vi "Shooter Button SUBVI.vi"   [LabVIEW 2011]
types:
  T1 = cluster{"Digital Input [1-16][0]":bool, "Digital Input [1-16][1]":bool, "Digital Input [1-16][2]":bool, "Digital Input [1-16][3]":bool, "Digital Input [1-16][4]":bool, "Digital Input [1-16][5]":bool, "Digital Input [1-16][6]":bool, "Digital Input [1-16][7]":bool, "Digital Input [1-16][8]":bool, "Digital Input [1-16][9]":bool, "Digital Input [1-16][10]":bool, "Digital Input [1-16][11]":bool, "Digital Input [1-16][12]":bool, "Digital Input [1-16][13]":bool, "Digital Input [1-16][14]":bool, "Digital Input [1-16][15]":bool}
  T2 = typedef "WPI_DigitalInputDevRef.ctl" = cluster{"DevStatus":errorcluster, "DIO Channel":T3, "Digital Module":T4}
  T3 = typedef "FPGA_DIOChannel.ctl" = enum8{"DIO 1", "DIO 2", "DIO 3", "DIO 4", "DIO 5", "DIO 6", "DIO 7", "DIO 8", "DIO 9", "DIO 10", "DIO 11", "DIO 12", "DIO 13", "DIO 14", "Invalid"}
  T4 = typedef "FPGA_TypedefDigitalModule.ctl" = enum16{"Digital Module 1", "Digital Module 2"}
  T5 = typedef "WPI_MotorControlDeviceRef.ctl" = cluster{"DeviceStatus":errorcluster, "Type":enum16{"PWM", "CAN"}, "PWM":cluster{"Digital Module":T4, "PWM Channel":T6, "DeadBand":T7}, "CAN":cluster{"Device Number":u8, "Control Mode":T8, "Semaphore":T9, "Max Vout":dbl}, "Invert":bool, "TransformRef":T10, "InvTransformRef":T10}
  T6 = typedef "FPGA_DIOPWMChannel.ctl" = enum8{"PWM 1", "PWM 2", "PWM 3", "PWM 4", "PWM 5", "PWM 6", "PWM 7", "PWM 8", "PWM 9", "PWM 10", "Invalid"}
  T7 = typedef "WPI_PWMDeadband.ctl" = cluster{"Name":string, "maxPositivePwm":i32, "minPositivePwm":i32, "centerPwm":i32, "maxNegativePwm":i32, "minNegativePwm":i32, "angularRange":u16}
  T8 = typedef "WPI_CANJaguar_ControlMode.ctl" = enum8{"Percent VBus", "Current", "Speed", "Position", "Voltage"}
  T9 = typedef "Semaphore RefNum" = refnum<k1>
  T10 = typedef "WPI_PWMTransform_ConPane.ctl" = refnum<vi>
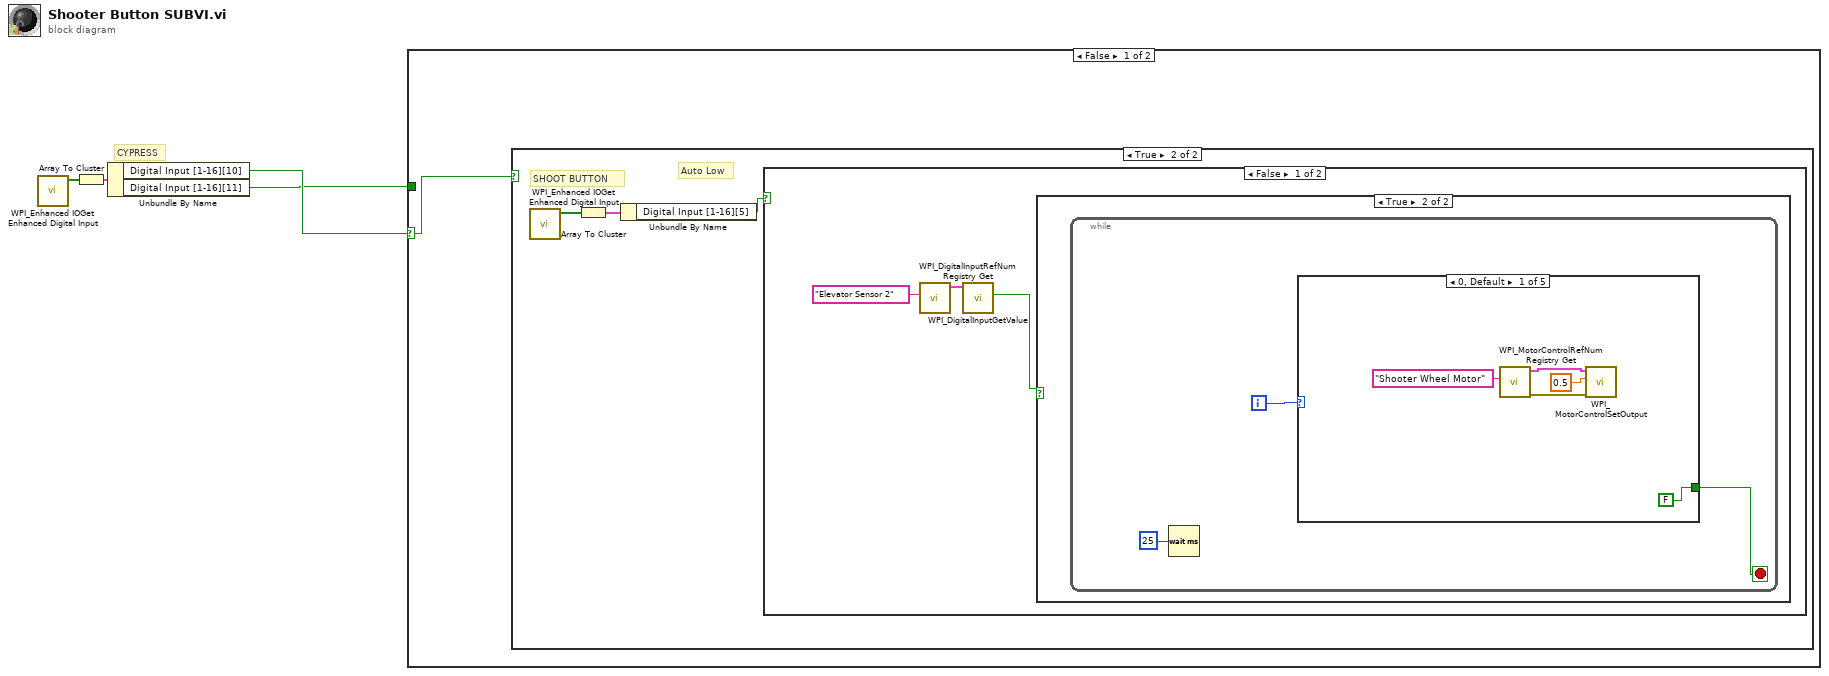
[diagram p0: block diagram]
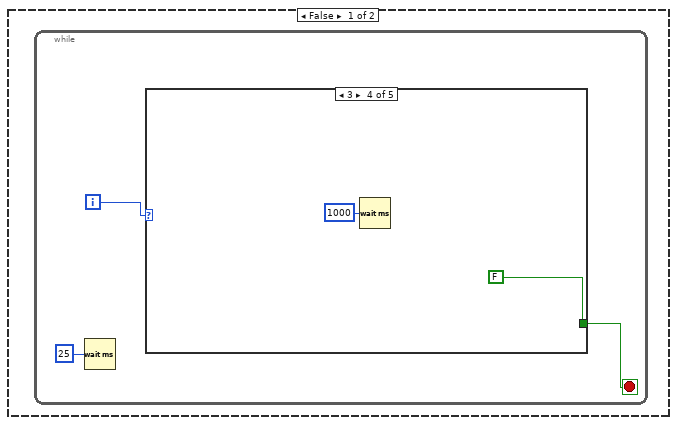
[diagram p3: hidden frame]
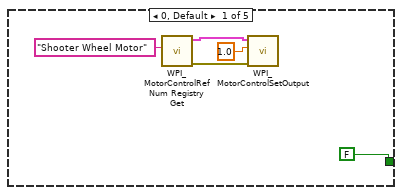
[diagram p4: hidden frame]
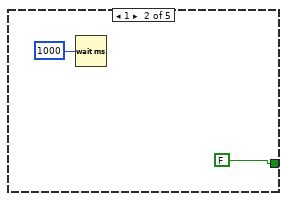
[diagram p5: hidden frame]
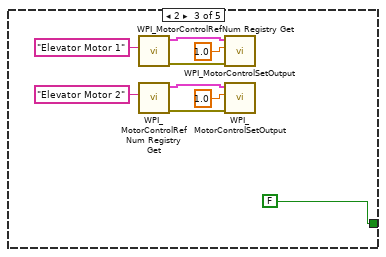
[diagram p6: hidden frame]
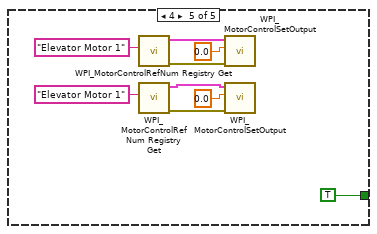
[diagram p7: hidden frame]
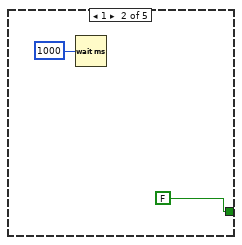
[diagram p8: hidden frame]
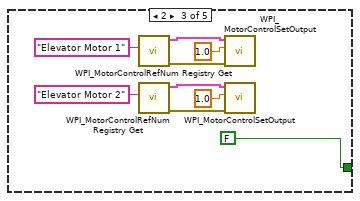
[diagram p9: hidden frame]
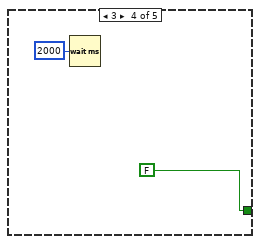
[diagram p10: hidden frame]
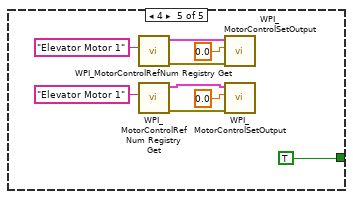
[diagram p11: hidden frame]
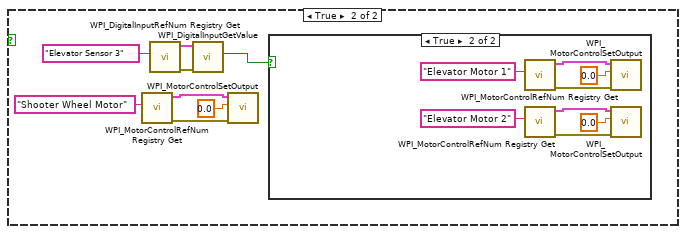
[diagram p12: hidden frame]
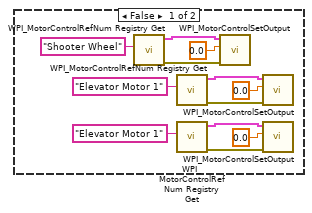
[diagram p13: hidden frame]
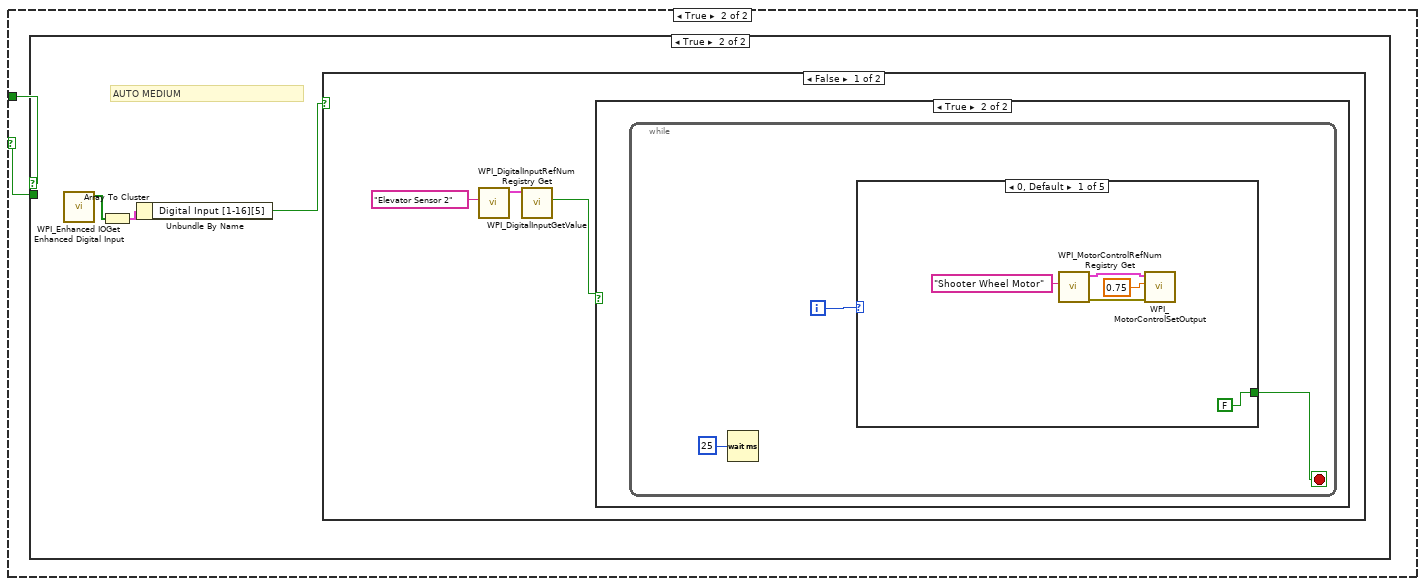
[diagram p14: hidden frame]
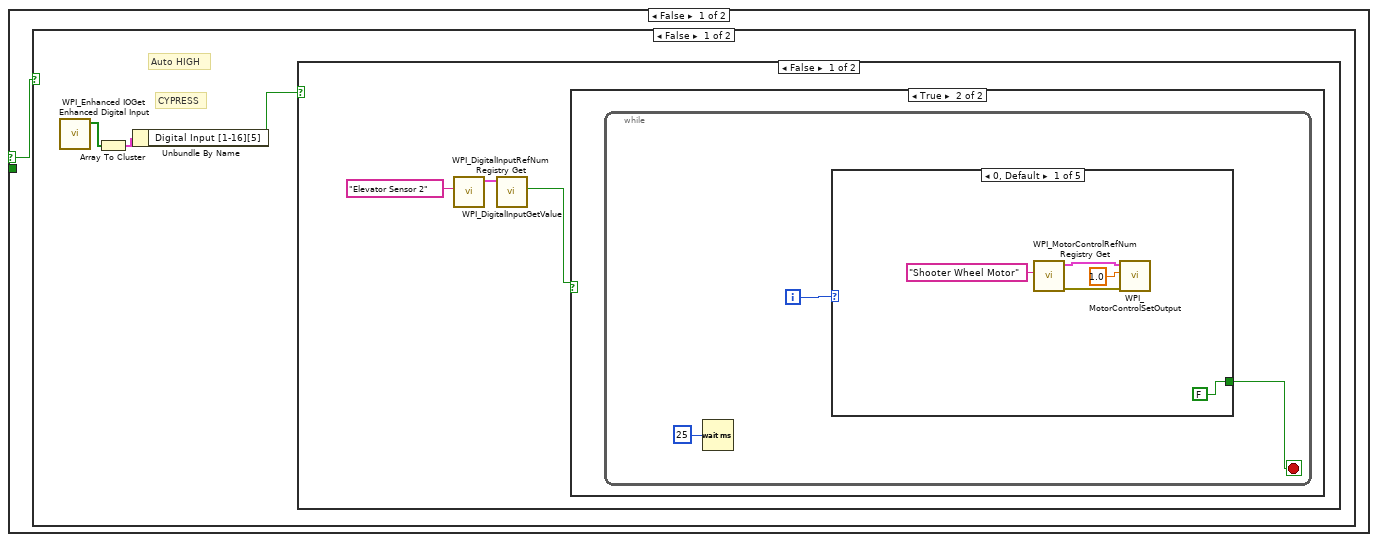
[diagram p15: hidden frame]
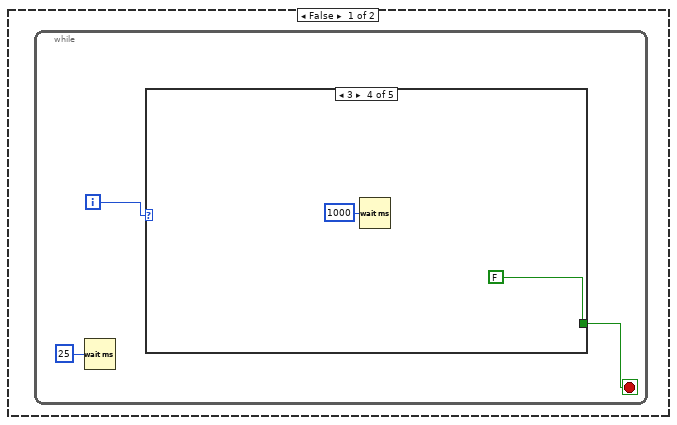
[diagram p16: hidden frame]
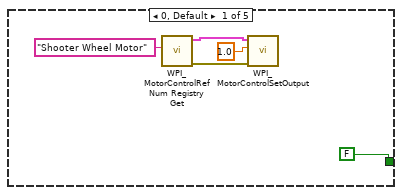
[diagram p17: hidden frame]
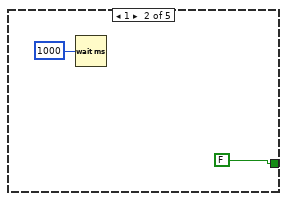
[diagram p18: hidden frame]
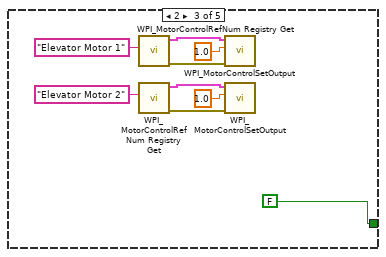
[diagram p19: hidden frame]
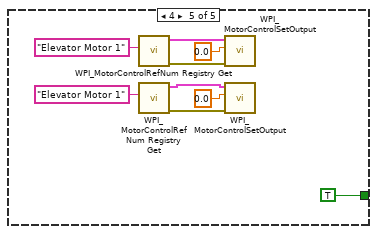
[diagram p20: hidden frame]
diagram:
  # "CYPRESS"
  n1 = call <vilib>:"WPI_Enhanced IOGet Enhanced Digital Input.vi"() -> ("Digital Input [1-16]"=w4:bool[])  [unwired: 10 in, 1 out]
  n2 = Array To Cluster(array=w4) -> (cluster=w3:T1)
  n3 = Unbundle By Name(w3) -> ("Digital Input [1-16][10]"=w2:bool, "Digital Input [1-16][11]"=w1:bool)
  n4 = case shown="False" w2 {
    selector: w2 -> [w5 w100]
    tunnel: w1 -> [_ w101]
    frame False {
      n5 = case shown="True" w5 {
        frame False {
        }
        frame True {
          # "Auto Low"
          # "SHOOT BUTTON"
          n6 = call <vilib>:"WPI_Enhanced IOGet Enhanced Digital Input.vi"() -> ("Digital Input [1-16]"=w8:bool[])  [unwired: 10 in, 1 out]
          n7 = Array To Cluster(array=w8) -> (cluster=w7:T1)
          n8 = Unbundle By Name(w7) -> ("Digital Input [1-16][5]"=w6:bool)
          n9 = case shown="False" w6 {
            frame False {
              n10 = call <vilib>:"WPI_DigitalInputRefNum Registry Get.vi"("refnum name"="Elevator Sensor 2") -> ("DigitalInputDevRef"=w10:T2)  [unwired: 9 in, 1 out]
              n11 = call <vilib>:"WPI_DigitalInputGetValue.vi"("DigitalInputDevRef"=w10) -> ("Value"=w9:bool)  [unwired: 8 in, 2 out]
              n12 = case shown="True" w9 {
                frame False {
                  n13 = while {
                    i -> [w14]
                    stop <- w12 stop-if-true
                    n14 = Wait (ms)(milliseconds to wait=u32 25) -> ()  [unwired: 1 out]
                    n15 = case shown="3" w14 {
                      tunnel: [FALSE FALSE FALSE FALSE TRUE] -> w12
                      frame 0, Default {
                        n16 = call <vilib>:"WPI_MotorControlRefNum Registry Get.vi"("refnum name"="Shooter Wheel Motor") -> ("error out"=w19:errorcluster, "MotorControlDevRef"=w18:T5)  [unwired: 9 in]
                        n17 = call <vilib>:"WPI_MotorControlSetOutput.vi"("error in (no error)"=w19, "Output"=1.0, "MotorControlDevRef"=w18) -> ()  [unwired: 7 in, 2 out]
                      }
                      frame 1 {
                        n18 = Wait (ms)(milliseconds to wait=u32 1000) -> ()  [unwired: 1 out]
                      }
                      frame 2 {
                        n19 = call <vilib>:"WPI_MotorControlRefNum Registry Get.vi"("refnum name"="Elevator Motor 1") -> ("error out"=w26:errorcluster, "MotorControlDevRef"=w25:T5)  [unwired: 9 in]
                        n20 = call <vilib>:"WPI_MotorControlRefNum Registry Get.vi"("refnum name"="Elevator Motor 2") -> ("error out"=w30:errorcluster, "MotorControlDevRef"=w29:T5)  [unwired: 9 in]
                        n21 = call <vilib>:"WPI_MotorControlSetOutput.vi"("error in (no error)"=w26, "Output"=1.0, "MotorControlDevRef"=w25) -> ()  [unwired: 7 in, 2 out]
                        n22 = call <vilib>:"WPI_MotorControlSetOutput.vi"("error in (no error)"=w30, "Output"=1.0, "MotorControlDevRef"=w29) -> ()  [unwired: 7 in, 2 out]
                      }
                      frame 3 {
                        n23 = Wait (ms)(milliseconds to wait=1000) -> ()  [unwired: 1 out]
                      }
                      frame 4 {
                        n24 = call <vilib>:"WPI_MotorControlRefNum Registry Get.vi"("refnum name"="Elevator Motor 1") -> ("error out"=w39:errorcluster, "MotorControlDevRef"=w34:T5)  [unwired: 9 in]
                        n25 = call <vilib>:"WPI_MotorControlRefNum Registry Get.vi"("refnum name"="Elevator Motor 1") -> ("error out"=w35:errorcluster, "MotorControlDevRef"=w36:T5)  [unwired: 9 in]
                        n26 = call <vilib>:"WPI_MotorControlSetOutput.vi"("error in (no error)"=w39, "Output"=0.0, "MotorControlDevRef"=w34) -> ()  [unwired: 7 in, 2 out]
                        n27 = call <vilib>:"WPI_MotorControlSetOutput.vi"("error in (no error)"=w35, "Output"=0.0, "MotorControlDevRef"=w36) -> ()  [unwired: 7 in, 2 out]
                      }
                    }
                  }
                }
                frame True {
                  n28 = while {
                    i -> [w44]
                    stop <- w42 stop-if-true
                    n29 = Wait (ms)(milliseconds to wait=u32 25) -> ()  [unwired: 1 out]
                    n30 = case shown="0, Default" w44 {
                      tunnel: [FALSE FALSE FALSE FALSE TRUE] -> w42
                      frame 0, Default {
                        n31 = call <vilib>:"WPI_MotorControlRefNum Registry Get.vi"("refnum name"="Shooter Wheel Motor") -> ("error out"=w49:errorcluster, "MotorControlDevRef"=w48:T5)  [unwired: 9 in]
                        n32 = call <vilib>:"WPI_MotorControlSetOutput.vi"("error in (no error)"=w49, "Output"=0.5, "MotorControlDevRef"=w48) -> ()  [unwired: 7 in, 2 out]
                      }
                      frame 1 {
                        n33 = Wait (ms)(milliseconds to wait=u32 1000) -> ()  [unwired: 1 out]
                      }
                      frame 2 {
                        n34 = call <vilib>:"WPI_MotorControlRefNum Registry Get.vi"("refnum name"="Elevator Motor 1") -> ("error out"=w56:errorcluster, "MotorControlDevRef"=w55:T5)  [unwired: 9 in]
                        n35 = call <vilib>:"WPI_MotorControlRefNum Registry Get.vi"("refnum name"="Elevator Motor 2") -> ("error out"=w60:errorcluster, "MotorControlDevRef"=w59:T5)  [unwired: 9 in]
                        n36 = call <vilib>:"WPI_MotorControlSetOutput.vi"("error in (no error)"=w56, "Output"=1.0, "MotorControlDevRef"=w55) -> ()  [unwired: 7 in, 2 out]
                        n37 = call <vilib>:"WPI_MotorControlSetOutput.vi"("error in (no error)"=w60, "Output"=1.0, "MotorControlDevRef"=w59) -> ()  [unwired: 7 in, 2 out]
                      }
                      frame 3 {
                        n38 = Wait (ms)(milliseconds to wait=2000) -> ()  [unwired: 1 out]
                      }
                      frame 4 {
                        n39 = call <vilib>:"WPI_MotorControlRefNum Registry Get.vi"("refnum name"="Elevator Motor 1") -> ("error out"=w69:errorcluster, "MotorControlDevRef"=w63:T5)  [unwired: 9 in]
                        n40 = call <vilib>:"WPI_MotorControlRefNum Registry Get.vi"("refnum name"="Elevator Motor 1") -> ("error out"=w65:errorcluster, "MotorControlDevRef"=w66:T5)  [unwired: 9 in]
                        n41 = call <vilib>:"WPI_MotorControlSetOutput.vi"("error in (no error)"=w69, "Output"=0.0, "MotorControlDevRef"=w63) -> ()  [unwired: 7 in, 2 out]
                        n42 = call <vilib>:"WPI_MotorControlSetOutput.vi"("error in (no error)"=w65, "Output"=0.0, "MotorControlDevRef"=w66) -> ()  [unwired: 7 in, 2 out]
                      }
                    }
                  }
                }
              }
            }
            frame True {
              n43 = call <vilib>:"WPI_MotorControlRefNum Registry Get.vi"("refnum name"="Shooter Wheel Motor") -> ("error out"=w75:errorcluster, "MotorControlDevRef"=w74:T5)  [unwired: 9 in]
              n44 = call <vilib>:"WPI_DigitalInputRefNum Registry Get.vi"("refnum name"="Elevator Sensor 3") -> ("error out"=w78:errorcluster, "DigitalInputDevRef"=w77:T2)  [unwired: 9 in]
              n45 = call <vilib>:"WPI_DigitalInputGetValue.vi"("error in (no error)"=w78, "DigitalInputDevRef"=w77) -> ("Value"=w76:bool)  [unwired: 7 in, 2 out]
              n46 = call <vilib>:"WPI_MotorControlSetOutput.vi"("error in (no error)"=w75, "Output"=0.0, "MotorControlDevRef"=w74) -> ()  [unwired: 7 in, 2 out]
              n47 = case shown="True" w76 {
                frame False {
                  n48 = call <vilib>:"WPI_MotorControlRefNum Registry Get.vi"("refnum name"="Shooter Wheel") -> ("error out"=w83:errorcluster, "MotorControlDevRef"=w82:T5)  [unwired: 9 in]
                  n49 = call <vilib>:"WPI_MotorControlRefNum Registry Get.vi"("refnum name"="Elevator Motor 1") -> ("error out"=w87:errorcluster, "MotorControlDevRef"=w86:T5)  [unwired: 9 in]
                  n50 = call <vilib>:"WPI_MotorControlRefNum Registry Get.vi"("refnum name"="Elevator Motor 1") -> ("error out"=w91:errorcluster, "MotorControlDevRef"=w90:T5)  [unwired: 9 in]
                  n51 = call <vilib>:"WPI_MotorControlSetOutput.vi"("error in (no error)"=w83, "Output"=0.0, "MotorControlDevRef"=w82) -> ()  [unwired: 7 in, 2 out]
                  n52 = call <vilib>:"WPI_MotorControlSetOutput.vi"("error in (no error)"=w87, "Output"=0.0, "MotorControlDevRef"=w86) -> ()  [unwired: 7 in, 2 out]
                  n53 = call <vilib>:"WPI_MotorControlSetOutput.vi"("error in (no error)"=w91, "Output"=0.0, "MotorControlDevRef"=w90) -> ()  [unwired: 7 in, 2 out]
                }
                frame True {
                  n54 = call <vilib>:"WPI_MotorControlRefNum Registry Get.vi"("refnum name"="Elevator Motor 1") -> ("error out"=w95:errorcluster, "MotorControlDevRef"=w94:T5)  [unwired: 9 in]
                  n55 = call <vilib>:"WPI_MotorControlRefNum Registry Get.vi"("refnum name"="Elevator Motor 2") -> ("error out"=w99:errorcluster, "MotorControlDevRef"=w98:T5)  [unwired: 9 in]
                  n56 = call <vilib>:"WPI_MotorControlSetOutput.vi"("error in (no error)"=w95, "Output"=0.0, "MotorControlDevRef"=w94) -> ()  [unwired: 7 in, 2 out]
                  n57 = call <vilib>:"WPI_MotorControlSetOutput.vi"("error in (no error)"=w99, "Output"=0.0, "MotorControlDevRef"=w98) -> ()  [unwired: 7 in, 2 out]
                }
              }
            }
          }
        }
      }
    }
    frame True {
      n58 = case shown="True" w101 {
        selector: w101 -> [w102 _]
        tunnel: w100 -> [_ _]
        frame False {
          n59 = case shown="False" w102 {
            frame False {
              # "CYPRESS"
              # "Auto HIGH"
              n60 = call <vilib>:"WPI_Enhanced IOGet Enhanced Digital Input.vi"() -> ("Digital Input [1-16]"=w105:bool[])  [unwired: 10 in, 1 out]
              n61 = Array To Cluster(array=w105) -> (cluster=w104:T1)
              n62 = Unbundle By Name(w104) -> ("Digital Input [1-16][5]"=w103:bool)
              n63 = case shown="False" w103 {
                frame False {
                  n64 = call <vilib>:"WPI_DigitalInputRefNum Registry Get.vi"("refnum name"="Elevator Sensor 2") -> ("DigitalInputDevRef"=w107:T2)  [unwired: 9 in, 1 out]
                  n65 = call <vilib>:"WPI_DigitalInputGetValue.vi"("DigitalInputDevRef"=w107) -> ("Value"=w106:bool)  [unwired: 8 in, 2 out]
                  n66 = case shown="True" w106 {
                    frame False {
                      n67 = while {
                        i -> [w111]
                        stop <- w109 stop-if-true
                        n68 = Wait (ms)(milliseconds to wait=u32 25) -> ()  [unwired: 1 out]
                        n69 = case shown="3" w111 {
                          tunnel: [FALSE FALSE FALSE FALSE TRUE] -> w109
                          frame 0, Default {
                            n70 = call <vilib>:"WPI_MotorControlRefNum Registry Get.vi"("refnum name"="Shooter Wheel Motor") -> ("error out"=w116:errorcluster, "MotorControlDevRef"=w115:T5)  [unwired: 9 in]
                            n71 = call <vilib>:"WPI_MotorControlSetOutput.vi"("error in (no error)"=w116, "Output"=1.0, "MotorControlDevRef"=w115) -> ()  [unwired: 7 in, 2 out]
                          }
                          frame 1 {
                            n72 = Wait (ms)(milliseconds to wait=u32 1000) -> ()  [unwired: 1 out]
                          }
                          frame 2 {
                            n73 = call <vilib>:"WPI_MotorControlRefNum Registry Get.vi"("refnum name"="Elevator Motor 1") -> ("error out"=w123:errorcluster, "MotorControlDevRef"=w122:T5)  [unwired: 9 in]
                            n74 = call <vilib>:"WPI_MotorControlRefNum Registry Get.vi"("refnum name"="Elevator Motor 2") -> ("error out"=w127:errorcluster, "MotorControlDevRef"=w126:T5)  [unwired: 9 in]
                            n75 = call <vilib>:"WPI_MotorControlSetOutput.vi"("error in (no error)"=w123, "Output"=1.0, "MotorControlDevRef"=w122) -> ()  [unwired: 7 in, 2 out]
                            n76 = call <vilib>:"WPI_MotorControlSetOutput.vi"("error in (no error)"=w127, "Output"=1.0, "MotorControlDevRef"=w126) -> ()  [unwired: 7 in, 2 out]
                          }
                          frame 3 {
                            n77 = Wait (ms)(milliseconds to wait=1000) -> ()  [unwired: 1 out]
                          }
                          frame 4 {
                            n78 = call <vilib>:"WPI_MotorControlRefNum Registry Get.vi"("refnum name"="Elevator Motor 1") -> ("error out"=w136:errorcluster, "MotorControlDevRef"=w131:T5)  [unwired: 9 in]
                            n79 = call <vilib>:"WPI_MotorControlRefNum Registry Get.vi"("refnum name"="Elevator Motor 1") -> ("error out"=w132:errorcluster, "MotorControlDevRef"=w133:T5)  [unwired: 9 in]
                            n80 = call <vilib>:"WPI_MotorControlSetOutput.vi"("error in (no error)"=w136, "Output"=0.0, "MotorControlDevRef"=w131) -> ()  [unwired: 7 in, 2 out]
                            n81 = call <vilib>:"WPI_MotorControlSetOutput.vi"("error in (no error)"=w132, "Output"=0.0, "MotorControlDevRef"=w133) -> ()  [unwired: 7 in, 2 out]
                          }
                        }
                      }
                    }
                    frame True {
                      n82 = while {
                        i -> [w141]
                        stop <- w139 stop-if-true
                        n83 = Wait (ms)(milliseconds to wait=u32 25) -> ()  [unwired: 1 out]
                        n84 = case shown="0, Default" w141 {
                          tunnel: [FALSE FALSE FALSE FALSE TRUE] -> w139
                          frame 0, Default {
                            n85 = call <vilib>:"WPI_MotorControlRefNum Registry Get.vi"("refnum name"="Shooter Wheel Motor") -> ("error out"=w146:errorcluster, "MotorControlDevRef"=w145:T5)  [unwired: 9 in]
                            n86 = call <vilib>:"WPI_MotorControlSetOutput.vi"("error in (no error)"=w146, "Output"=1.0, "MotorControlDevRef"=w145) -> ()  [unwired: 7 in, 2 out]
                          }
                          frame 1 {
                            n87 = Wait (ms)(milliseconds to wait=u32 1000) -> ()  [unwired: 1 out]
                          }
                          frame 2 {
                            n88 = call <vilib>:"WPI_MotorControlRefNum Registry Get.vi"("refnum name"="Elevator Motor 1") -> ("error out"=w153:errorcluster, "MotorControlDevRef"=w152:T5)  [unwired: 9 in]
                            n89 = call <vilib>:"WPI_MotorControlRefNum Registry Get.vi"("refnum name"="Elevator Motor 2") -> ("error out"=w157:errorcluster, "MotorControlDevRef"=w156:T5)  [unwired: 9 in]
                            n90 = call <vilib>:"WPI_MotorControlSetOutput.vi"("error in (no error)"=w153, "Output"=1.0, "MotorControlDevRef"=w152) -> ()  [unwired: 7 in, 2 out]
                            n91 = call <vilib>:"WPI_MotorControlSetOutput.vi"("error in (no error)"=w157, "Output"=1.0, "MotorControlDevRef"=w156) -> ()  [unwired: 7 in, 2 out]
                          }
                          frame 3 {
                            n92 = Wait (ms)(milliseconds to wait=2000) -> ()  [unwired: 1 out]
                          }
                          frame 4 {
                            n93 = call <vilib>:"WPI_MotorControlRefNum Registry Get.vi"("refnum name"="Elevator Motor 1") -> ("error out"=w166:errorcluster, "MotorControlDevRef"=w160:T5)  [unwired: 9 in]
                            n94 = call <vilib>:"WPI_MotorControlRefNum Registry Get.vi"("refnum name"="Elevator Motor 1") -> ("error out"=w162:errorcluster, "MotorControlDevRef"=w163:T5)  [unwired: 9 in]
                            n95 = call <vilib>:"WPI_MotorControlSetOutput.vi"("error in (no error)"=w166, "Output"=0.0, "MotorControlDevRef"=w160) -> ()  [unwired: 7 in, 2 out]
                            n96 = call <vilib>:"WPI_MotorControlSetOutput.vi"("error in (no error)"=w162, "Output"=0.0, "MotorControlDevRef"=w163) -> ()  [unwired: 7 in, 2 out]
                          }
                        }
                      }
                    }
                  }
                }
                frame True {
                  n97 = call <vilib>:"WPI_MotorControlRefNum Registry Get.vi"("refnum name"="Shooter Wheel Motor") -> ("error out"=w172:errorcluster, "MotorControlDevRef"=w171:T5)  [unwired: 9 in]
                  n98 = call <vilib>:"WPI_DigitalInputRefNum Registry Get.vi"("refnum name"="Elevator Sensor 3") -> ("error out"=w175:errorcluster, "DigitalInputDevRef"=w174:T2)  [unwired: 9 in]
                  n99 = call <vilib>:"WPI_DigitalInputGetValue.vi"("error in (no error)"=w175, "DigitalInputDevRef"=w174) -> ("Value"=w173:bool)  [unwired: 7 in, 2 out]
                  n100 = call <vilib>:"WPI_MotorControlSetOutput.vi"("error in (no error)"=w172, "Output"=0.0, "MotorControlDevRef"=w171) -> ()  [unwired: 7 in, 2 out]
                  n101 = case shown="True" w173 {
                    frame False {
                      n102 = call <vilib>:"WPI_MotorControlRefNum Registry Get.vi"("refnum name"="Shooter Wheel") -> ("error out"=w180:errorcluster, "MotorControlDevRef"=w179:T5)  [unwired: 9 in]
                      n103 = call <vilib>:"WPI_MotorControlRefNum Registry Get.vi"("refnum name"="Elevator Motor 1") -> ("error out"=w184:errorcluster, "MotorControlDevRef"=w183:T5)  [unwired: 9 in]
                      n104 = call <vilib>:"WPI_MotorControlRefNum Registry Get.vi"("refnum name"="Elevator Motor 1") -> ("error out"=w188:errorcluster, "MotorControlDevRef"=w187:T5)  [unwired: 9 in]
                      n105 = call <vilib>:"WPI_MotorControlSetOutput.vi"("error in (no error)"=w180, "Output"=0.0, "MotorControlDevRef"=w179) -> ()  [unwired: 7 in, 2 out]
                      n106 = call <vilib>:"WPI_MotorControlSetOutput.vi"("error in (no error)"=w184, "Output"=0.0, "MotorControlDevRef"=w183) -> ()  [unwired: 7 in, 2 out]
                      n107 = call <vilib>:"WPI_MotorControlSetOutput.vi"("error in (no error)"=w188, "Output"=0.0, "MotorControlDevRef"=w187) -> ()  [unwired: 7 in, 2 out]
                    }
                    frame True {
                      n108 = call <vilib>:"WPI_MotorControlRefNum Registry Get.vi"("refnum name"="Elevator Motor 1") -> ("error out"=w192:errorcluster, "MotorControlDevRef"=w191:T5)  [unwired: 9 in]
                      n109 = call <vilib>:"WPI_MotorControlRefNum Registry Get.vi"("refnum name"="Elevator Motor 2") -> ("error out"=w196:errorcluster, "MotorControlDevRef"=w195:T5)  [unwired: 9 in]
                      n110 = call <vilib>:"WPI_MotorControlSetOutput.vi"("error in (no error)"=w192, "Output"=0.0, "MotorControlDevRef"=w191) -> ()  [unwired: 7 in, 2 out]
                      n111 = call <vilib>:"WPI_MotorControlSetOutput.vi"("error in (no error)"=w196, "Output"=0.0, "MotorControlDevRef"=w195) -> ()  [unwired: 7 in, 2 out]
                    }
                  }
                }
              }
            }
            frame True {
            }
          }
        }
        frame True {
          # "AUTO MEDIUM"
          n112 = call <vilib>:"WPI_Enhanced IOGet Enhanced Digital Input.vi"() -> ("Digital Input [1-16]"=w198:bool[])  [unwired: 10 in, 1 out]
          n113 = Array To Cluster(array=w198) -> (cluster=w199:T1)
          n114 = Unbundle By Name(w199) -> ("Digital Input [1-16][5]"=w197:bool)
          n115 = case shown="False" w197 {
            frame False {
              n116 = call <vilib>:"WPI_DigitalInputRefNum Registry Get.vi"("refnum name"="Elevator Sensor 2") -> ("DigitalInputDevRef"=w201:T2)  [unwired: 9 in, 1 out]
              n117 = call <vilib>:"WPI_DigitalInputGetValue.vi"("DigitalInputDevRef"=w201) -> ("Value"=w200:bool)  [unwired: 8 in, 2 out]
              n118 = case shown="True" w200 {
                frame False {
                  n119 = while {
                    i -> [w205]
                    stop <- w203 stop-if-true
                    n120 = Wait (ms)(milliseconds to wait=u32 25) -> ()  [unwired: 1 out]
                    n121 = case shown="3" w205 {
                      tunnel: [FALSE FALSE FALSE FALSE TRUE] -> w203
                      frame 0, Default {
                        n122 = call <vilib>:"WPI_MotorControlRefNum Registry Get.vi"("refnum name"="Shooter Wheel Motor") -> ("error out"=w210:errorcluster, "MotorControlDevRef"=w209:T5)  [unwired: 9 in]
                        n123 = call <vilib>:"WPI_MotorControlSetOutput.vi"("error in (no error)"=w210, "Output"=1.0, "MotorControlDevRef"=w209) -> ()  [unwired: 7 in, 2 out]
                      }
                      frame 1 {
                        n124 = Wait (ms)(milliseconds to wait=u32 1000) -> ()  [unwired: 1 out]
                      }
                      frame 2 {
                        n125 = call <vilib>:"WPI_MotorControlRefNum Registry Get.vi"("refnum name"="Elevator Motor 1") -> ("error out"=w217:errorcluster, "MotorControlDevRef"=w216:T5)  [unwired: 9 in]
                        n126 = call <vilib>:"WPI_MotorControlRefNum Registry Get.vi"("refnum name"="Elevator Motor 2") -> ("error out"=w221:errorcluster, "MotorControlDevRef"=w220:T5)  [unwired: 9 in]
                        n127 = call <vilib>:"WPI_MotorControlSetOutput.vi"("error in (no error)"=w217, "Output"=1.0, "MotorControlDevRef"=w216) -> ()  [unwired: 7 in, 2 out]
                        n128 = call <vilib>:"WPI_MotorControlSetOutput.vi"("error in (no error)"=w221, "Output"=1.0, "MotorControlDevRef"=w220) -> ()  [unwired: 7 in, 2 out]
                      }
                      frame 3 {
                        n129 = Wait (ms)(milliseconds to wait=1000) -> ()  [unwired: 1 out]
                      }
                      frame 4 {
                        n130 = call <vilib>:"WPI_MotorControlRefNum Registry Get.vi"("refnum name"="Elevator Motor 1") -> ("error out"=w230:errorcluster, "MotorControlDevRef"=w225:T5)  [unwired: 9 in]
                        n131 = call <vilib>:"WPI_MotorControlRefNum Registry Get.vi"("refnum name"="Elevator Motor 1") -> ("error out"=w226:errorcluster, "MotorControlDevRef"=w227:T5)  [unwired: 9 in]
                        n132 = call <vilib>:"WPI_MotorControlSetOutput.vi"("error in (no error)"=w230, "Output"=0.0, "MotorControlDevRef"=w225) -> ()  [unwired: 7 in, 2 out]
                        n133 = call <vilib>:"WPI_MotorControlSetOutput.vi"("error in (no error)"=w226, "Output"=0.0, "MotorControlDevRef"=w227) -> ()  [unwired: 7 in, 2 out]
                      }
                    }
                  }
                }
                frame True {
                  n134 = while {
                    i -> [w235]
                    stop <- w233 stop-if-true
                    n135 = Wait (ms)(milliseconds to wait=u32 25) -> ()  [unwired: 1 out]
                    n136 = case shown="0, Default" w235 {
                      tunnel: [FALSE FALSE FALSE FALSE TRUE] -> w233
                      frame 0, Default {
                        n137 = call <vilib>:"WPI_MotorControlRefNum Registry Get.vi"("refnum name"="Shooter Wheel Motor") -> ("error out"=w240:errorcluster, "MotorControlDevRef"=w239:T5)  [unwired: 9 in]
                        n138 = call <vilib>:"WPI_MotorControlSetOutput.vi"("error in (no error)"=w240, "Output"=0.75, "MotorControlDevRef"=w239) -> ()  [unwired: 7 in, 2 out]
                      }
                      frame 1 {
                        n139 = Wait (ms)(milliseconds to wait=u32 1000) -> ()  [unwired: 1 out]
                      }
                      frame 2 {
                        n140 = call <vilib>:"WPI_MotorControlRefNum Registry Get.vi"("refnum name"="Elevator Motor 1") -> ("error out"=w247:errorcluster, "MotorControlDevRef"=w246:T5)  [unwired: 9 in]
                        n141 = call <vilib>:"WPI_MotorControlRefNum Registry Get.vi"("refnum name"="Elevator Motor 2") -> ("error out"=w251:errorcluster, "MotorControlDevRef"=w250:T5)  [unwired: 9 in]
                        n142 = call <vilib>:"WPI_MotorControlSetOutput.vi"("error in (no error)"=w247, "Output"=1.0, "MotorControlDevRef"=w246) -> ()  [unwired: 7 in, 2 out]
                        n143 = call <vilib>:"WPI_MotorControlSetOutput.vi"("error in (no error)"=w251, "Output"=1.0, "MotorControlDevRef"=w250) -> ()  [unwired: 7 in, 2 out]
                      }
                      frame 3 {
                        n144 = Wait (ms)(milliseconds to wait=2000) -> ()  [unwired: 1 out]
                      }
                      frame 4 {
                        n145 = call <vilib>:"WPI_MotorControlRefNum Registry Get.vi"("refnum name"="Elevator Motor 1") -> ("error out"=w260:errorcluster, "MotorControlDevRef"=w254:T5)  [unwired: 9 in]
                        n146 = call <vilib>:"WPI_MotorControlRefNum Registry Get.vi"("refnum name"="Elevator Motor 1") -> ("error out"=w256:errorcluster, "MotorControlDevRef"=w257:T5)  [unwired: 9 in]
                        n147 = call <vilib>:"WPI_MotorControlSetOutput.vi"("error in (no error)"=w260, "Output"=0.0, "MotorControlDevRef"=w254) -> ()  [unwired: 7 in, 2 out]
                        n148 = call <vilib>:"WPI_MotorControlSetOutput.vi"("error in (no error)"=w256, "Output"=0.0, "MotorControlDevRef"=w257) -> ()  [unwired: 7 in, 2 out]
                      }
                    }
                  }
                }
              }
            }
            frame True {
              n149 = call <vilib>:"WPI_MotorControlRefNum Registry Get.vi"("refnum name"="Shooter Wheel Motor") -> ("error out"=w266:errorcluster, "MotorControlDevRef"=w265:T5)  [unwired: 9 in]
              n150 = call <vilib>:"WPI_DigitalInputRefNum Registry Get.vi"("refnum name"="Elevator Sensor 3") -> ("error out"=w269:errorcluster, "DigitalInputDevRef"=w268:T2)  [unwired: 9 in]
              n151 = call <vilib>:"WPI_DigitalInputGetValue.vi"("error in (no error)"=w269, "DigitalInputDevRef"=w268) -> ("Value"=w267:bool)  [unwired: 7 in, 2 out]
              n152 = call <vilib>:"WPI_MotorControlSetOutput.vi"("error in (no error)"=w266, "Output"=0.0, "MotorControlDevRef"=w265) -> ()  [unwired: 7 in, 2 out]
              n153 = case shown="True" w267 {
                frame False {
                  n154 = call <vilib>:"WPI_MotorControlRefNum Registry Get.vi"("refnum name"="Shooter Wheel") -> ("error out"=w274:errorcluster, "MotorControlDevRef"=w273:T5)  [unwired: 9 in]
                  n155 = call <vilib>:"WPI_MotorControlRefNum Registry Get.vi"("refnum name"="Elevator Motor 1") -> ("error out"=w278:errorcluster, "MotorControlDevRef"=w277:T5)  [unwired: 9 in]
                  n156 = call <vilib>:"WPI_MotorControlRefNum Registry Get.vi"("refnum name"="Elevator Motor 1") -> ("error out"=w282:errorcluster, "MotorControlDevRef"=w281:T5)  [unwired: 9 in]
                  n157 = call <vilib>:"WPI_MotorControlSetOutput.vi"("error in (no error)"=w274, "Output"=0.0, "MotorControlDevRef"=w273) -> ()  [unwired: 7 in, 2 out]
                  n158 = call <vilib>:"WPI_MotorControlSetOutput.vi"("error in (no error)"=w278, "Output"=0.0, "MotorControlDevRef"=w277) -> ()  [unwired: 7 in, 2 out]
                  n159 = call <vilib>:"WPI_MotorControlSetOutput.vi"("error in (no error)"=w282, "Output"=0.0, "MotorControlDevRef"=w281) -> ()  [unwired: 7 in, 2 out]
                }
                frame True {
                  n160 = call <vilib>:"WPI_MotorControlRefNum Registry Get.vi"("refnum name"="Elevator Motor 1") -> ("error out"=w286:errorcluster, "MotorControlDevRef"=w285:T5)  [unwired: 9 in]
                  n161 = call <vilib>:"WPI_MotorControlRefNum Registry Get.vi"("refnum name"="Elevator Motor 2") -> ("error out"=w290:errorcluster, "MotorControlDevRef"=w289:T5)  [unwired: 9 in]
                  n162 = call <vilib>:"WPI_MotorControlSetOutput.vi"("error in (no error)"=w286, "Output"=0.0, "MotorControlDevRef"=w285) -> ()  [unwired: 7 in, 2 out]
                  n163 = call <vilib>:"WPI_MotorControlSetOutput.vi"("error in (no error)"=w290, "Output"=0.0, "MotorControlDevRef"=w289) -> ()  [unwired: 7 in, 2 out]
                }
              }
            }
          }
        }
      }
    }
  }
